vi "NACA_0015_Pressure.vi"(3 "Mode":T5, 5 "Traverse line In":T1 {"Row Duration (mins)" format="%#.1f"; "Row No" min=0; "Trace Gas Concentration (%)" min=0.0 format="%#.2f"; "Emission Rate (l/min)" format="%#.2f"; "Tunnel Speed" format="%#.2f"; "Start X" format="%#.2f"; "Start Y" format="%#.2f"; "Start Z" format="%#.2f"; "End X" format="%#.2f"; "End Y" format="%#.2f"; "End Z" format="%#.2f"; "Averaging time (min)" min=0.0 format="%#.2f"}) -> (0 "Error Message":string, 1 "Status":T4, 2 "Traverse line Out":T1 {"Row Duration (mins)" format="%#.1f"; "Row No" min=0; "Trace Gas Concentration (%)" min=0.0 format="%#.2f"; "Emission Rate (l/min)" format="%#.2f"; "Tunnel Speed" format="%#.2f"; "Start X" format="%#.2f"; "Start Y" format="%#.2f"; "Start Z" format="%#.2f"; "End X" format="%#.2f"; "End Y" format="%#.2f"; "End Z" format="%#.2f"; "Averaging time (min)" min=0.0 format="%#.2f"})   [LabVIEW 2011]
uses:
  Gen Trav/Traverse_cluster.ctl
  Gen Trav/Spacing.ctl
  Controls/Multi_run_mode.ctl
  Controls/User_Specific_mode.ctl
  Gen Trav/Multi_Run_Status.ctl
  Controls/Save_Data.ctl
  Controls/Setup.ctl
  <vilib>/Analysis/1siggen.llb/Ramp Pattern by Delta.vi
  Globals/Extra_Commands_Global.vi
  Globals/Meas_global.vi
  <vilib>/Analysis/NI_AALBase.lvlib
panel:
  in  "stop":bool
  out "XY Graph":cluster{dbl[], dbl[]}(graph)
  out "Measurement No":i32
  # "X           Y            Z"
  # "Start"
  # "End"
  # "X           Y            Z"
  # "Start"
  # "End"
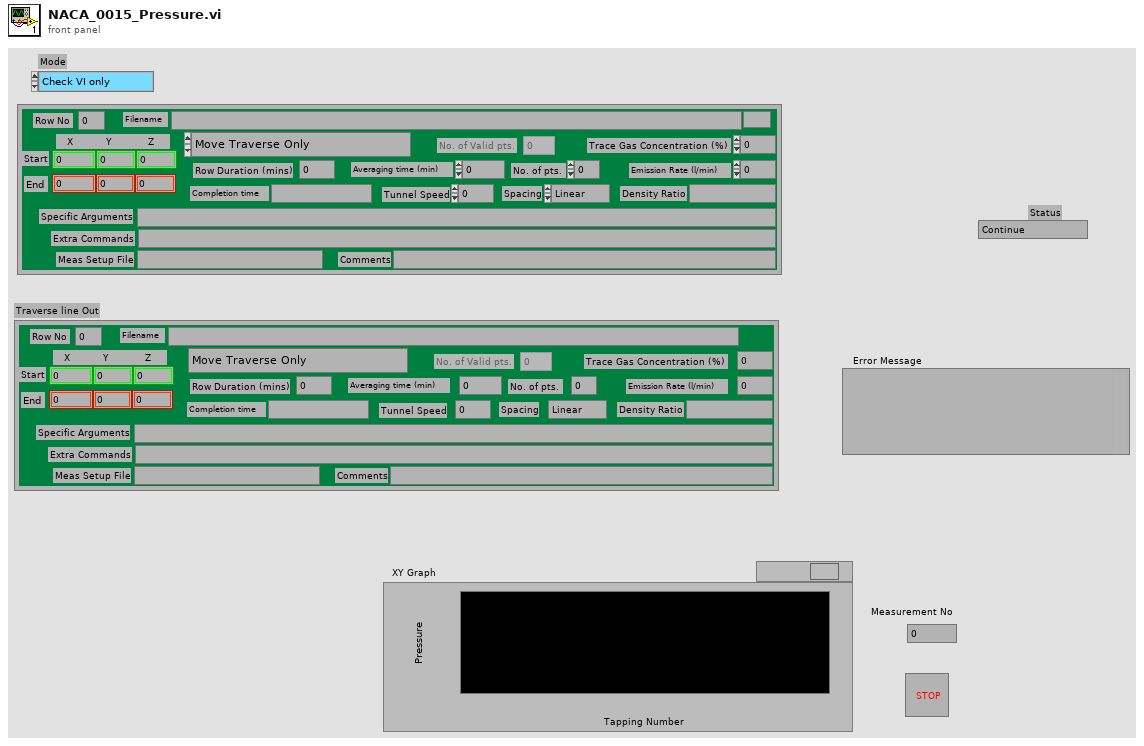
[diagram p1: front panel]
types:
  T1 = typedef "Traverse_cluster.ctl" = cluster{"Start X":dbl, "Start Y":dbl, "Start Z":dbl, "End X":dbl, "End Y":dbl, "End Z":dbl, "No. of pts.":i32, "Spacing":T2, "Filename":path, "Tunnel Speed":dbl, "Averaging time (min)":dbl, "Extra Commands":string, "Specific Arguments":string, "Emission Rate (l/min)":dbl, "Trace Gas Concentration (%)":dbl, "Density Ratio":string, "Comments":string, "Row No":i32, "Row Type Selector":T3, "Completion time":string, "Row Duration (mins)":dbl, "No. of Valid pts.":i32, "Meas Setup File":string}
  T2 = typedef "Spacing.ctl" = enum16{"Linear", "Log", "Gauss", "Specified", "N/A"}
  T3 = typedef "Multi_run_mode.ctl" = enum16{"Move Traverse Only", "Set Tunnel Speed Only", "Set Source Only", "Set Measurement Conditions", "Single Measurement", "Vertical Profile", "Lateral Profile", "Longitudinal Profile", "Explore Volume", "Multi-Axis Profile", "Auto Calibrate", "Meas Fast FID Bkgnd", "Check Beam Power", "Scanning Valve Measurement", "Run VI Named:", "Set ADAM Ch", "Wait (minutes)", "Send Message", "Synchronize With:", "Fall Back to this Row", "Turn Off Row Repeating", "Blank Row", "Traverse 3D Volume"}
  T4 = typedef "Multi_Run_Status.ctl" = enum16{"Continue", "Jump to Next Point", "Jump to Next Row", "Jump To Fall Back", "Terminate Run"}
  T5 = typedef "User_Specific_mode.ctl" = enum16{"Check VI only", "Run VI"}
  T6 = typedef "Save_Data.ctl" = enum16{"Save No Data", "Save Data"}
  T7 = typedef "Setup.ctl" = enum16{"Run Program", "Show Setup", "Save Current Setup", "Setup Front Panel"}
  T8 = typedef "Status_Cluster.ctl" = cluster{"Status":T4, "Error Type":string, "Error Description":string}
  T9 = typedef "Analysis_info_cluster.ctl" = cluster{"Colour":u32, "Inst type":T10, "Inst name":string, "Symbol":string, "Code name":string, "Extra Info":string, "Inst Array":T11, "Extra Titles":string[], "Extra Values":string[], "Eng Values":dbl[], "Time (ms)":dbl[], "Voltage":dbl[], "U":dbl, "u^2":dbl, "u^3":dbl, "u^4":dbl, "Skew_u":dbl, "Kurt_u":dbl, "Sd Error in Mean":dbl, "% u'/U":dbl, "X":dbl, "Y":dbl, "Z":dbl, "Spectra":T12, "Autocorrelation":T12, "Timescale integral to 25%":dbl, "Sd Error in Variance":dbl, "Calib File":path, "Calib Constants":dbl[], "Histogram":T12, "Output Position":bool, "Full Stats":bool, "Weighting":dbl[], "Av Sampling Rate":dbl, "Av No of Samples":dbl, "Total Meas Time (s)":dbl}
  T10 = typedef "Inst_type.ctl" = enum16{"Propeller anemometer", "Raw voltage", "Pressure Transducer", "Pitot-static tube", "Preston tube", "Hot wire", "Cross wire 1", "Cross wire 2", "Generic Linear", "Generic Polynomial", "Generic BackPoly", "Fast FID", "Thermocouple", "Cold wire", "Pulsed Wire", "LDA Vel", "LDA Tran time", "LDA Arr time"}
  T11 = typedef "Instrument_Array.ctl" = enum16{"PWA", "LDA", "Analogue"}
  T12 = typedef "XY_Plot_Cluster.ctl" = cluster{"First Name":string, "Second Name":string, "X axis name":string, "Y axis name":string, "X array":dbl[], "Y array":dbl[]}
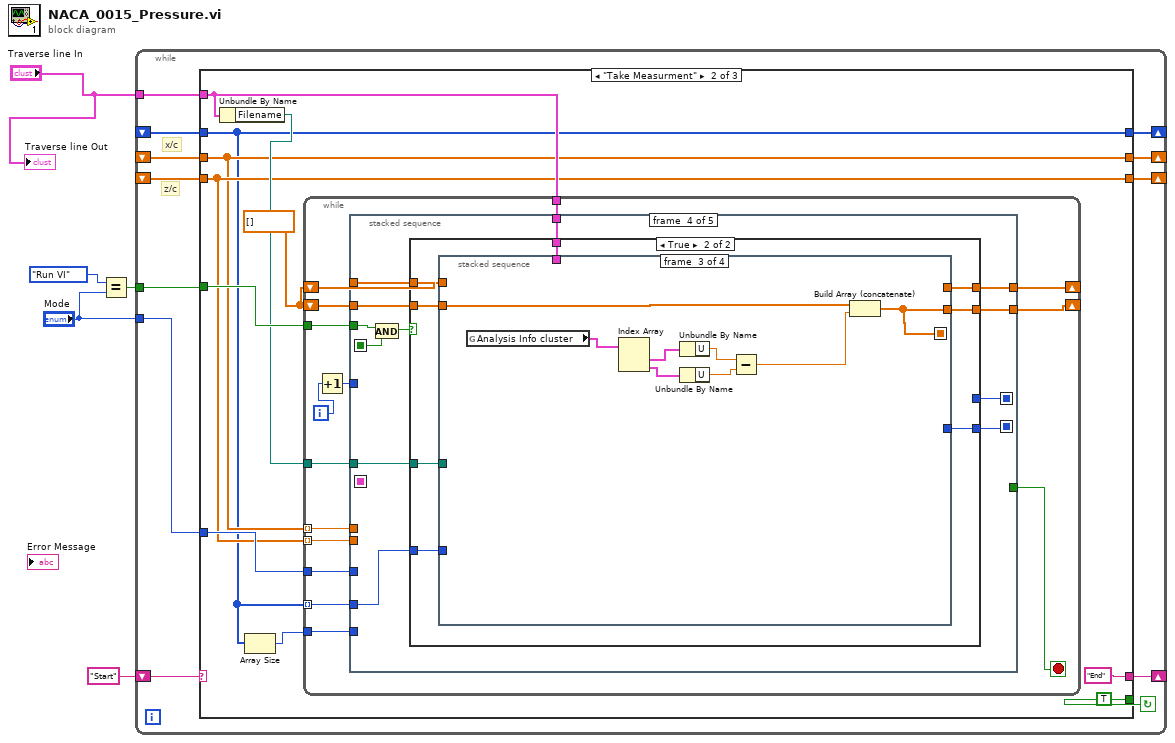
[diagram p0: block diagram]
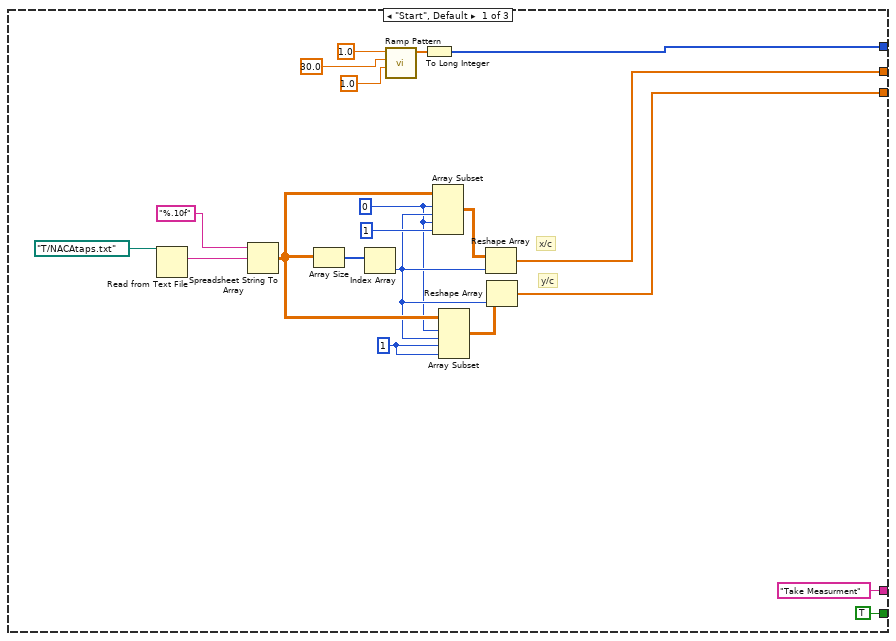
[diagram p2: hidden frame]
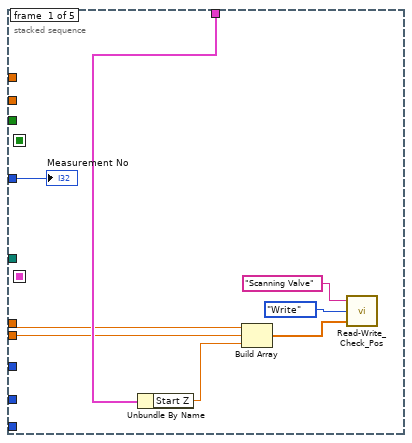
[diagram p3: hidden frame]
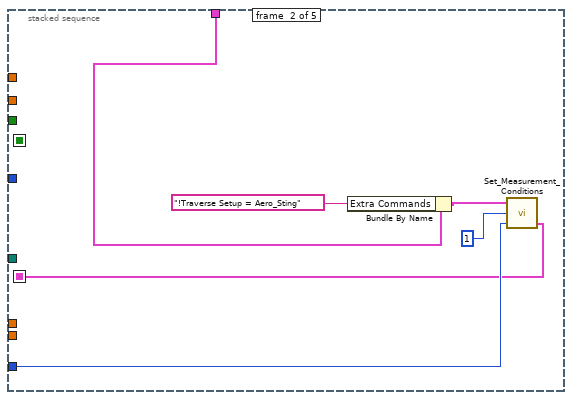
[diagram p4: hidden frame]
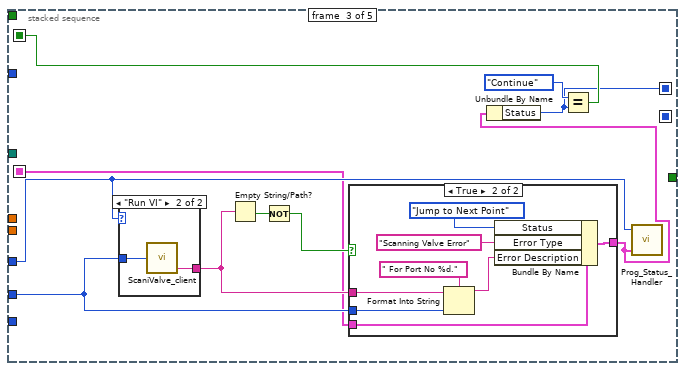
[diagram p5: hidden frame]
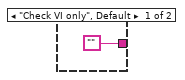
[diagram p6: hidden frame]
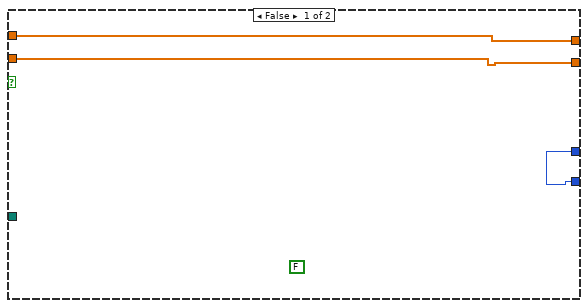
[diagram p8: hidden frame]
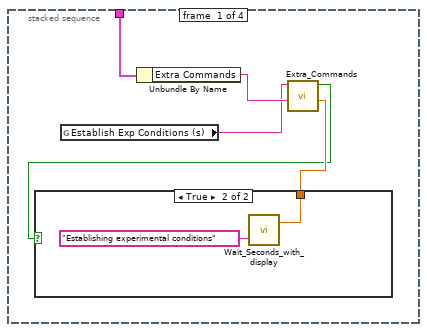
[diagram p9: hidden frame]
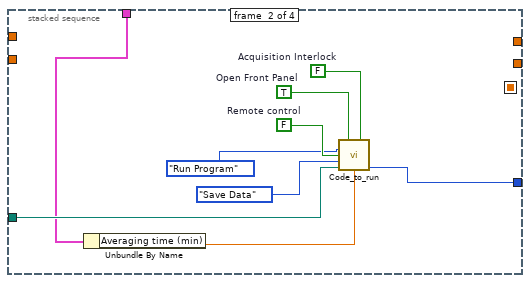
[diagram p11: hidden frame]
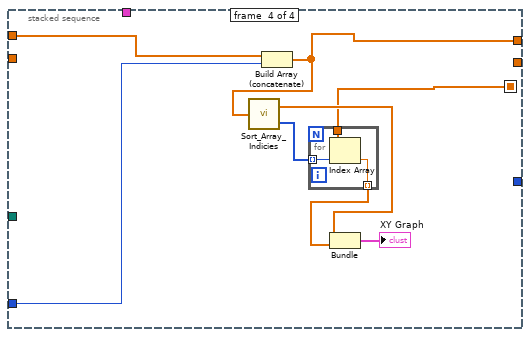
[diagram p12: hidden frame]
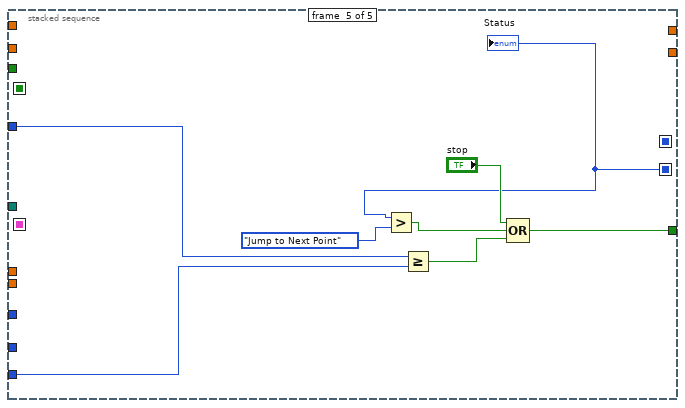
[diagram p13: hidden frame]
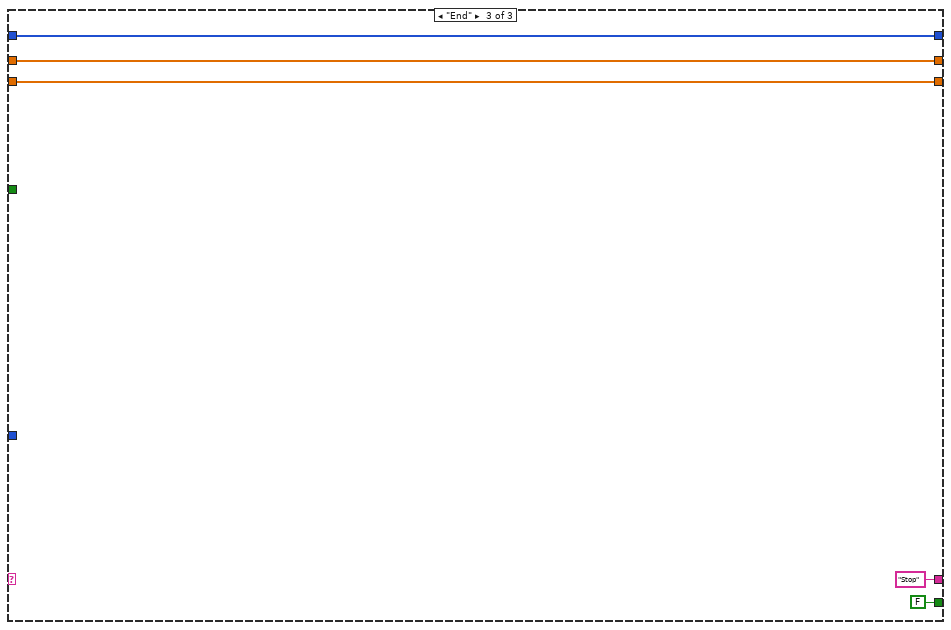
[diagram p14: hidden frame]
diagram:
  n1 = Equal?(x=User_Specific_mode."Run VI" ("Mode"), y="Mode") -> (x = y?=w2:bool)
  n2 = while {
    tunnel: "Traverse line In" -> [w16]
    shift-right: [w15] -> _
    shift-left: "Start" -> [w14]
    tunnel: "Mode" -> [w13]
    tunnel: w2 -> [w12]
    shift-right: [w11] -> _
    shift-left: _ -> [w10]
    shift-right: [w9] -> _
    shift-left: _ -> [w7]
    shift-right: [w8] -> _
    shift-left: _ -> [w6]
    stop <- w17 continue-if-true
    # "z/c"
    # "x/c"
    n3 = case shown="\"Take Measurment\"" w14 {
      tunnel: [TRUE TRUE FALSE] -> w17
      tunnel: w16 -> [_ w44 _]
      tunnel: ["Take Measurment" "End" "Stop"] -> w15
      tunnel: w13 -> [_ w42 _]
      tunnel: w12 -> [_ w45 _]
      tunnel: [w33 w39 w168] -> w11
      tunnel: w10 -> [_ w39 w168]
      tunnel: [w19 w40 w167] -> w9
      tunnel: [w18 w41 w166] -> w8
      tunnel: w7 -> [_ w40 w167]
      tunnel: w6 -> [_ w41 w166]
      frame "Start", Default {
        w20 = 1 ("index")
        w21 = 0 ("index")
        # "y/c"
        # "x/c"
        n4 = Read from Text File(file (use dialog)=path "T:/NACAtaps.txt") -> (text=w29:string)  [unwired: 3 in, 3 out]
        n5 = Spreadsheet String To Array(format string="%.10f", spreadsheet string=w29) -> (array=w25:dbl[][])  [unwired: 2 in]
        n6 = Array Size(array=w25) -> (size(s)=w27:i32[])
        n7 = Index Array(array=w27) -> (element=w22:i32)  [unwired: 1 in]
        n8 = call-poly <vilib>:"Ramp Pattern.vi"("start"=1.0, "end"=30.0, "delta"=1.0) -> ("Ramp Pattern"=w37:dbl[])  [unwired: 6 in, 2 out]
        n9 = To Long Integer(number=w37) -> (32bit integer=w33:i32[])
        n10 = Array Subset(array=w25, index (row)=w21, length (row)=w22, index (col)=w21, length (col)=1 ("length")) -> (w24:dbl[][])
        n11 = Array Subset(array=w25, index (row)=w21, length (row)=w22, index (col)=w20, length (col)=w20) -> (w23:dbl[][])
        n12 = Reshape Array(w24, w22) -> (w19:dbl[])
        n13 = Reshape Array(w23, w22) -> (w18:dbl[])
      }
      frame "Take Measurment" {
        w46 = dbl[] []
        n14 = Unbundle By Name(w44) -> ("Filename"=w43:path)
        n15 = Array Size(array=w39) -> (size(s)=w38:i32)
        n16 = while {
          tunnel: w42 -> [w58]
          tunnel: w45 -> [w55]
          tunnel: w43 -> [w63]
          shift-right: [w61] -> _
          shift-left: w46 -> [w62]
          shift-right: [w59] -> _
          shift-left: w46 -> [w60]
          tunnel: w44 -> [w57]
          tunnel: w39 -> [w52] mode=indexing
          tunnel: w40 -> [w51] mode=indexing
          tunnel: w41 -> [w50] mode=indexing
          tunnel: w38 -> [w49]
          i -> [w54]
          stop <- w56 stop-if-true
          n17 = Increment(x=w54) -> (x+1=w53:i32)
          n18 = stacked-sequence {
            seq-local: [_ _ w81 _ _] -> [_ _ _ w103 _]
            seq-local: [_ _ w80 _ _] -> [_ _ _ w104 _]
            seq-local: [_ _ _ w105 _] -> [_ _ _ _ w159]
            seq-local: [_ w72 _ _ _] -> [_ _ w78 _ _]
            tunnel: w63 -> [_ _ _ w111 _]
            tunnel: w62 -> [_ _ _ w110 _]
            tunnel: [_ _ _ w109 _] -> w61
            tunnel: w60 -> [_ _ _ w108 _]
            tunnel: [_ _ _ w107 _] -> w59
            tunnel: w58 -> [_ w73 w84 _ _]
            tunnel: w57 -> [w70 w74 _ w106 _]
            tunnel: w53 -> [w71 _ _ _ w162]
            tunnel: [_ _ _ _ w160] -> w56
            tunnel: w55 -> [_ _ _ w102 _]
            tunnel: w52 -> [_ _ w79 w100 _]
            tunnel: w51 -> [w69 _ _ _ _]
            tunnel: w50 -> [w68 _ _ _ _]
            tunnel: w49 -> [_ _ _ _ w158]
            frame #0 {
              n19 = Unbundle By Name(w70) -> ("Start Z"=w67:dbl)
              n20 = Build Array(w69, w68, w67) -> (w66:dbl[])
              n21 = call "Read-Write_Check_Pos.vi"("Position input"=w66, "Mode"=enum16{"Read", "Write"}."Write", "Traverse Name"="Scanning Valve") -> ()  [unwired: 1 out]
              "Measurement No" <- w71
            }
            frame #1 {
              n22 = Bundle By Name(cluster=w74, "Extra Commands"="!Traverse Setup = Aero_Sting") -> (w77:T1)
              n23 = call "Set_Measurement_Conditions.vi"("Simulate/Run"=w73, "Currently on Point"=1, "Traverse line"=w77) -> ("Status Cluster"=w72:T8)  [unwired: 2 in]
            }
            frame #2 {
              n24 = case shown="\"Run VI\"" w84 {
                tunnel: w79 -> [_ w90]
                tunnel: ["" w89] -> w85
                frame "Check VI only", Default {
                }
                frame "Run VI" {
                  n25 = call "ScaniValve_client.vi"("Port Number"=w90) -> ("Error String"=w89:string)  [unwired: 2 out]
                }
              }
              n26 = Empty String/Path?(string/path=w85) -> (empty?=w87:bool)
              n27 = Not(x=w87) -> (.not. x?=w86:bool)
              n28 = case shown="True" w86 {
                tunnel: w78 -> [w91 w99]
                tunnel: [w91 w96] -> w82
                tunnel: w85 -> [_ w93]
                tunnel: w79 -> [_ w92]
                frame False {
                }
                frame True {
                  n29 = Format Into String(format string=" For Port No %d." ("Format String"), initial string=w93, w92) -> (resulting string=w94:string)  [unwired: 1 in, 1 out]
                  n30 = Bundle By Name(cluster=w99, "Status"=Multi_Run_Status."Jump to Next Point", "Error Type"="Scanning Valve Error" ("t"), "Error Description"=w94) -> (w96:T8)
                }
              }
              n31 = Unbundle By Name(w82) -> ("Status"=w80:T4)
              n32 = Equal?(x=Multi_Run_Status."Continue" ("Status"), y=w80) -> (x = y?=w81:bool)
              n33 = call "Prog_Status_Handler.vi"("Status Cluster"=w82, "Simulate/Run"=w84) -> ()  [unwired: 2 out]
            }
            frame #3 {
              n34 = And(x=w102, y=w103) -> (x .and. y?=w101:bool)
              n35 = case shown="True" w101 {
                tunnel: [w112 w122] -> w105
                tunnel: w111 -> [_ w121]
                tunnel: w110 -> [w114 w120]
                tunnel: [w114 w119] -> w109
                tunnel: w108 -> [w113 w118]
                tunnel: [w113 w117] -> w107
                tunnel: w106 -> [_ w116]
                tunnel: w100 -> [_ w115]
                tunnel: w104 -> [w112 _]
                frame False {
                  (unwired) FALSE ("stop")
                }
                frame True {
                  n36 = stacked-sequence {
                    seq-local: [_ _ w145 _] -> [_ _ _ w149]
                    tunnel: [_ w132 _ _] -> w122
                    tunnel: w121 -> [_ w131 _ _]
                    tunnel: w120 -> [_ _ w146 _]
                    tunnel: [_ _ w145 _] -> w119
                    tunnel: w118 -> [_ _ _ w154]
                    tunnel: [_ _ _ w152] -> w117
                    tunnel: w116 -> [w127 w130 _ _]
                    tunnel: w115 -> [_ _ _ w147]
                    frame #0 {
                      n37 = global read "Extra_Commands_Global.vi" "Establish Exp Conditions (s)"() -> (w124:string)
                      n38 = Unbundle By Name(w127) -> ("Extra Commands"=w126:string)
                      n39 = call "Extra_Commands.vi"("String to Search"=w126, "Command"=w124) -> ("Numeric Value"=w125:dbl, "Command Found"=w123:bool)  [unwired: 2 in, 2 out]
                      n40 = case shown="True" w123 {
                        tunnel: w125 -> [_ w129]
                        frame False {
                        }
                        frame True {
                          n41 = call "Wait_Seconds_with_display.vi"("Message"="Establishing experimental conditions", "Seconds to wait"=w129) -> ()  [unwired: 1 in, 1 out]
                        }
                      }
                    }
                    frame #1 {
                      w135 = FALSE  # Acquisition Interlock
                      w136 = TRUE  # Open Front Panel
                      w138 = FALSE  # Remote control
                      n42 = Unbundle By Name(w130) -> ("Averaging time (min)"=w137:dbl)
                      n43 = call "Code_to_run.vi"("Open Front Panel"=w136, "Acquisition Interlock"=w135, "setup"=Setup."Run Program", "Remote control"=w138, "File"=Save_Data."Save Data", "Results Filename"=w131, "Averaging time (min)"=w137) -> ("Status"=w132:T4)  [unwired: 4 in, 4 out]
                    }
                    frame #2 {
                      n44 = global read "Meas_global.vi" "Analysis Info cluster"() -> (w144:T9[])
                      n45 = Index Array(array=w144) -> (element #1=w143:T9, element #2=w142:T9)  [unwired: 2 in]
                      n46 = Unbundle By Name(w143) -> ("U"=w140:dbl)
                      n47 = Unbundle By Name(w142) -> ("U"=w139:dbl)
                      n48 = Subtract(x=w140, y=w139) -> (x-y=w141:dbl)
                      n49 = Build Array (concatenate)(w146, w141) -> (w145:dbl[])
                    }
                    frame #3 {
                      n50 = Build Array (concatenate)(w154, w147) -> (w152:dbl[])
                      n51 = call "Sort_Array_Indicies.vi"("unsorted array"=w152) -> ("sorted array"=w151:dbl[], "Sort Index"=w150:i32[])
                      n52 = for {
                        tunnel: w150 -> [w157] mode=indexing
                        tunnel: w149 -> [w156]
                        tunnel: [w155] -> w148 mode=indexing
                        n53 = Index Array(array=w156, index=w157) -> (element=w155:dbl)
                      }
                      n54 = Bundle("sorted array"=w151, w148) -> (→"XY Graph":cluster{"sorted array":dbl[], dbl[]})  [unwired: 1 out]
                    }
                  }
                }
              }
            }
            frame #4 {
              n55 = Greater?(x=w159, y=Multi_Run_Status."Jump to Next Point" ("Status")) -> (0:w164:bool)
              n56 = Greater Or Equal?(x=w162, y=w158) -> (x >= y?=w163:bool)
              n57 = Compound Arithmetic op=OR("stop", w164, w163) -> (w160:bool)
              "Status" <- w159
            }
          }
        }
      }
      frame "End" {
      }
    }
  }
  "Traverse line Out" <- "Traverse line In"
